vi "PZT Set Position-精调-信号灯.vi"(8 "Set Position （°/mm）":dbl, 9 "Origin":dbl=123.091, 10 "Range":dbl=335.57, 11 "Instrument":T1={"325 Resource "="GPIB0::13::INSTR", "Input (0:A) 325"=0, "Heater Output (1:1) 325"=1, "340 Resource"="GPIB0::14::INSTR", "Input (0:A) 340"=0, "Loop (0: 1)"=0, "Input (0:B) 340"=1, "Loop (1: 1)"=0, "340 Status"=refnum, "Instrument Type"=enum."PPMS-Rotate", "quantum design"=refnum, "semaphore 325"=refnum, "TCP master instance"=refnum, "M24C Resource"="GPIB0::24::INSTR", "4G supply"="GPIB0::24::INSTR", "Temp Status 24C"=refnum, "Temp"=refnum, "9T信号"=refnum, "limit"={"Field limit"=0.0, "Field rate limit"=0.0, "Temp limit"=0.0, "Temp low limit"=0.0, "Temp rate limit "=0.0}, "4g supply status"=refnum, "vi路径"="", "in-plane"="", "out-plane"="", "in-plane signal"=FALSE, "out-plane signal"=FALSE, "in plane 信号"=refnum, "pzt volt"=refnum, "Aborting"=refnum, "数据文件"=refnum, "warning"=refnum, "750 visa"="", "750 rotate"="", "335 Status 2"=refnum, "335 Resource "="GPIB0::24::INSTR", "Input (0:A) 335"=0, "Input (0:B) 335"=1, "Heater Output (1:1) 335"=1, "semaphore 340"=refnum, "semaphore 335"=refnum, "325 Status"=refnum, "semaphore 750"=refnum, "750 field status"=refnum, "camg 振荡状态"=refnum, "列表框"=refnum, "编辑列表框？"=refnum, "camg Rate"=refnum, "行数"=refnum, "TM620"="TCPIP0::192.168.1.5::4266::SOCKET"} {"Loop (1: 1)" items=["1"=1, "2"=2]; "Loop (0: 1)" items=["1"=1, "2"=2]; "Input (0:B) 340" items=["A", "B", "C", "D"]; "Heater Output (1:1) 335" items=["1"=1, "2"=2]; "Input (0:B) 335" items=["A", "B"]; "Input (0:A) 335" items=["A", "B"]; "Heater Output (1:1) 325" items=["1"=1, "2"=2]; "Input (0:A) 325" items=["A", "B"]; "Input (0:A) 340" items=["1"=1, "2"=2]}) -> (1 "Set Position-Real （°/mm）":dbl, 2 "Current Position （mm  /  °）":dbl)   [LabVIEW 2019, in "User lib.lvlib"]
uses:
  User lib.lvlib
  ctl/Instrument.ctl
  <vilib>/NI/Modbus Library/API/Master/Modbus Master.lvclass
  ctl/335 state.ctl
  ctl/Instrument Type.ctl
  C:/Users/fuyang/Desktop/postdoctor/labview/labview-measure/lib/QDInstrument.dll
  lib/QDInstrument.dll
  ctl/limit.ctl
  ctl/9T mag field stauts.ctl
  ctl/warning.ctl
panel:
  out "初始运动方向":bool
  out "x > 0?":bool
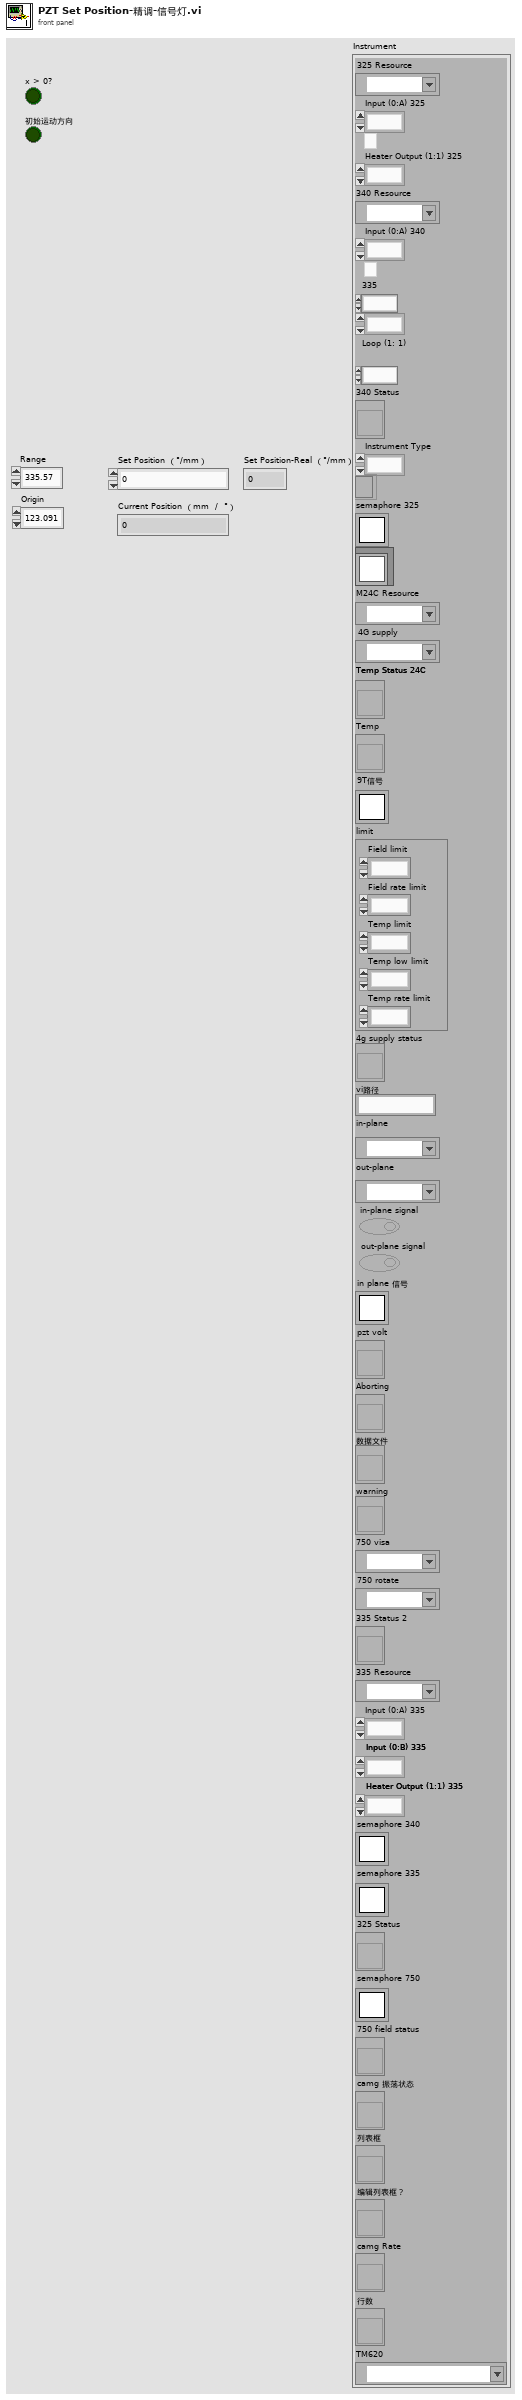
[diagram p1: front panel]
types:
  T1 = typedef "Instrument.ctl" = cluster{"325 Resource ":refnum<visa-resource-name>, "Input (0:A) 325":u16, "Heater Output (1:1) 325":u16, "340 Resource":refnum<visa-resource-name>, "Input (0:A) 340":u16, "Loop (0: 1)":u16, "Input (0:B) 340":u16, "Loop (1: 1)":u16, "340 Status":refnum<vi>, "Instrument Type":T2, "quantum design":refnum<k24>, "semaphore 325":T3, "TCP master instance":refnum<class "Modbus Master.lvclass">, "M24C Resource":refnum<visa-resource-name>, "4G supply":refnum<visa-resource-name>, "Temp Status 24C":refnum<vi>, "Temp":refnum<vi>, "9T信号":T3, "limit":T4, "4g supply status":refnum<vi>, "vi路径":string, "in-plane":refnum<visa-resource-name>, "out-plane":refnum<visa-resource-name>, "in-plane signal":bool, "out-plane signal":bool, "in plane 信号":T3, "pzt volt":refnum<vi>, "Aborting":refnum<vi>, "数据文件":refnum<vi>, "warning":refnum<vi>, "750 visa":refnum<visa-resource-name>, "750 rotate":refnum<visa-resource-name>, "335 Status 2":refnum<vi>, "335 Resource ":refnum<visa-resource-name>, "Input (0:A) 335":u16, "Input (0:B) 335":u16, "Heater Output (1:1) 335":u16, "semaphore 340":T3, "semaphore 335":T3, "325 Status":refnum<vi>, "semaphore 750":T3, "750 field status":refnum<vi>, "camg 振荡状态":refnum<vi>, "列表框":refnum<vi>, "编辑列表框？":refnum<vi>, "camg Rate":refnum<vi>, "行数":refnum<vi>, "TM620":refnum<visa-resource-name>}
  T2 = typedef "Instrument Type.ctl" = enum16{"PPMS", "VersaLab", "DynaCool", "SVSM", "PPMS-Rotate", "Lakeshore335", "lengtou2", "9T mag old", "9T cmag", "9T cmag DAC", "9T cmag rotate", "test"}
  T3 = typedef "Semaphore RefNum" = refnum<k1>
  T4 = typedef "limit.ctl" = cluster{"Field limit":dbl, "Field rate limit":dbl, "Temp limit":dbl, "Temp low limit":dbl, "Temp rate limit ":dbl}
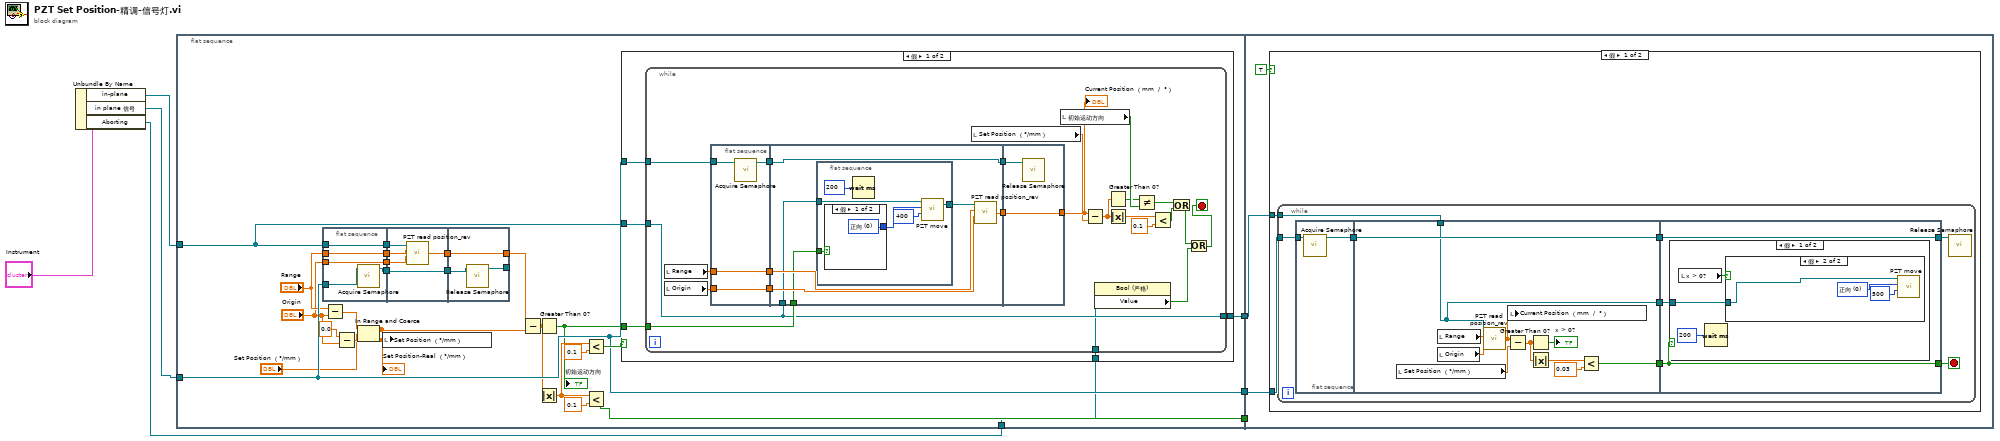
[diagram p0: block diagram]
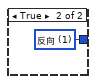
[diagram p2: hidden frame]
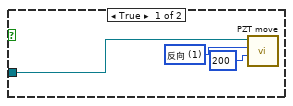
[diagram p4: hidden frame]
diagram:
  n1 = Unbundle By Name("Instrument") -> ("in-plane"=w4:refnum<visa-resource-name>, "in plane 信号"=w2:T3, "Aborting"=w1:refnum<vi>)
  n2 = flat-sequence {
    tunnel: [w31] -> w7
    tunnel: [w30] -> w6
    tunnel: w2 -> [w31]
    tunnel: w4 -> [w10]
    tunnel: [w9] -> w3
    tunnel: w1 -> [w8]
    tunnel: w7 -> [w98]
    tunnel: w6 -> [_]
    tunnel: w3 -> [w96]
    frame #0 {
      n3 = flat-sequence {
        tunnel: "Origin" -> [w35]
        tunnel: "Range" -> [w36]
        tunnel: w10 -> [w37]
        tunnel: [w37] -> w29
        tunnel: [w36] -> w28
        tunnel: [w35] -> w27
        tunnel: w31 -> [w34]
        tunnel: [w33] -> w26
        tunnel: w29 -> [w42]
        tunnel: w28 -> [w40]
        tunnel: w27 -> [w39]
        tunnel: [w41] -> w25
        tunnel: [w38] -> w24
        tunnel: w26 -> [w38]
        tunnel: [w45] -> w23
        tunnel: w25 -> [w45]
        tunnel: w24 -> [w44]
        tunnel: [w43] -> _
        frame #0 {
          n4 = call <vilib>:"Acquire Semaphore.vi"("semaphore"=w34) -> ("semaphore out"=w33:T3)  [unwired: 4 in, 2 out]
        }
        frame #1 {
          n5 = call "PZT read position_rev.vi"("Origin"=w39, "Range"=w40, "VISA resource name"=w42) -> ("Current Position （mm  /  °）"=w41:dbl)  [unwired: 1 in, 2 out]
        }
        frame #2 {
          n6 = call <vilib>:"Release Semaphore.vi"("semaphore"=w44) -> ("semaphore out"=w43:T3)  [unwired: 5 in, 1 out]
        }
      }
      n7 = Subtract(x="Range", y="Origin") -> (x-y=w19:dbl)
      n8 = Subtract(x=0.0, y="Origin") -> (x-y=w18:dbl)
      n9 = In Range and Coerce(upper limit=w19, x="Set Position （°/mm）", lower limit=w18) -> (coerced(x)=w16:dbl)  [unwired: 1 out]
      "Set Position-Real （°/mm）" <- w16
      n10 = local write "Set Position （°/mm）"(w16) -> ()
      n11 = Subtract(x=w23, y=w16) -> (x-y=w21:dbl)
      n12 = Greater Than 0?(x=w21) -> (x > 0?=w11:bool)
      "初始运动方向" <- w11
      n13 = Absolute Value(x=w21) -> (abs(x)=w13:dbl)
      n14 = Less?(x=w13, y=0.1) -> (x < y?=w32:bool)
      n15 = Less?(x=w13, y=0.1) -> (x < y?=w30:bool)
      n16 = case shown="假" w32 {
        tunnel: w31 -> [w50 _]
        tunnel: w11 -> [w49 _]
        tunnel: w10 -> [w48 w95]
        tunnel: [w47 w95] -> w9
        tunnel: w8 -> [w46 _]
        frame False {
          n17 = while {
            tunnel: w50 -> [w57]
            tunnel: w49 -> [w56]
            tunnel: w48 -> [w55]
            tunnel: [w55] -> w47
            tunnel: w46 -> [w54]
            stop <- w51 stop-if-true
            n18 = local read "Range"() -> (w73:dbl)
            n19 = local read "Origin"() -> (w72:dbl)
            n20 = flat-sequence {
              tunnel: w72 -> [w76]
              tunnel: w73 -> [w77]
              tunnel: [w77] -> w61
              tunnel: [w76] -> w60
              tunnel: [w75] -> w58
              tunnel: w57 -> [w74]
              tunnel: [w82] -> w62
              tunnel: w61 -> [w84]
              tunnel: w60 -> [w83]
              tunnel: [w81] -> w59
              tunnel: w58 -> [w81]
              tunnel: w55 -> [w80]
              tunnel: w56 -> [w79]
              tunnel: [w94] -> w71
              tunnel: w62 -> [w94]
              tunnel: w59 -> [w93]
              frame #0 {
                n21 = call <vilib>:"Acquire Semaphore.vi"("semaphore"=w74) -> ("semaphore out"=w75:T3)  [unwired: 4 in, 2 out]
              }
              frame #1 {
                n22 = flat-sequence {
                  tunnel: w80 -> [w90]
                  tunnel: [w88] -> w78
                  tunnel: w79 -> [w87]
                  frame #0 {
                    n23 = case shown="假" w87 {
                      tunnel: [w91 w92] -> w86
                      frame False {
                        w91 = u16 0 items=["正向", "反向"] ("移动方向")
                      }
                      frame True {
                        w92 = u16 1 items=["正向", "反向"] ("移动方向")
                      }
                    }
                    n24 = Wait (ms)(milliseconds to wait=u32 200 ("等待时间（毫秒）")) -> ()  [unwired: 1 out]
                    n25 = call "PZT move.vi"("移动步数"=400, "移动方向"=w86, "VISA resource name"=w90) -> ("VISA资源名称输出"=w88:refnum<visa-resource-name>)  [unwired: 1 in, 1 out]
                  }
                }
                n26 = call "PZT read position_rev.vi"("Origin"=w83, "Range"=w84, "VISA resource name"=w78) -> ("Current Position （mm  /  °）"=w82:dbl)  [unwired: 1 in, 2 out]
              }
              frame #2 {
                n27 = call <vilib>:"Release Semaphore.vi"("semaphore"=w93) -> ()  [unwired: 5 in, 2 out]
              }
            }
            n28 = local read "Set Position （°/mm）"() -> (w70:dbl)
            n29 = local read "初始运动方向"() -> (w66:bool)
            n30 = Subtract(x=w71, y=w70) -> (x-y=w67:dbl)
            n31 = property class="Bool (严格)"(reference=w54) -> ("Value"=w52:bool)  [unwired: 1 in, 2 out]
            n32 = Greater Than 0?(x=w67) -> (x > 0?=w65:bool)
            n33 = Absolute Value(x=w67) -> (abs(x)=w69:dbl)
            n34 = Not Equal?(x=w65, y=w66) -> (x != y?=w64:bool)
            n35 = Less?(x=w69, y=0.1) -> (x < y?=w63:bool)
            n36 = Or(x=w64, y=w63) -> (x .or. y?=w53:bool)
            n37 = Or(x=w53, y=w52) -> (x .or. y?=w51:bool)
            "Current Position （mm  /  °）" <- w71
          }
        }
        frame True {
        }
      }
    }
    frame #1 {
      n38 = case shown="假" TRUE {
        tunnel: w98 -> [w100 _]
        tunnel: w96 -> [w99 _]
        frame False {
          n39 = while {
            tunnel: w100 -> [w107]
            tunnel: w99 -> [w102]
            stop <- w108 stop-if-true
            n40 = flat-sequence {
              tunnel: [w110] -> w106
              tunnel: w107 -> [w109]
              tunnel: [w115] -> w105
              tunnel: w106 -> [w112]
              tunnel: [w112] -> w104
              tunnel: w102 -> [w111]
              tunnel: [w111] -> w101
              tunnel: [w123] -> w108
              tunnel: [w124] -> w103
              tunnel: w104 -> [w124]
              tunnel: w105 -> [w123]
              tunnel: w101 -> [w122]
              frame #0 {
                n41 = call <vilib>:"Acquire Semaphore.vi"("semaphore"=w109) -> ("semaphore out"=w110:T3)  [unwired: 4 in, 2 out]
              }
              frame #1 {
                n42 = local read "Set Position （°/mm）"() -> (w119:dbl)
                n43 = local read "Range"() -> (w121:dbl)
                n44 = local read "Origin"() -> (w120:dbl)
                n45 = call "PZT read position_rev.vi"("Origin"=w120, "Range"=w121, "VISA resource name"=w111) -> ("Current Position （mm  /  °）"=w113:dbl)  [unwired: 1 in, 2 out]
                n46 = Subtract(x=w113, y=w119) -> (x-y=w118:dbl)
                n47 = local write "Current Position （mm  /  °）"(w113) -> ()
                n48 = Greater Than 0?(x=w118) -> (x > 0?=→"x > 0?":bool)
                n49 = Absolute Value(x=w118) -> (abs(x)=w117:dbl)
                n50 = Less?(x=w117, y=0.03) -> (x < y?=w115:bool)
              }
              frame #2 {
                n51 = case shown="假" w123 {
                  tunnel: w122 -> [w125 _]
                  frame False {
                    n52 = local read "x > 0?"() -> (w127:bool)
                    n53 = Wait (ms)(milliseconds to wait=u32 200) -> ()  [unwired: 1 out]
                    n54 = case shown="假" w127 {
                      tunnel: w125 -> [w128 w131]
                      frame True {
                        w130 = u16 1 items=["正向", "反向"] ("移动方向")
                        n55 = call "PZT move.vi"("移动步数"=200, "移动方向"=w130, "VISA resource name"=w128) -> ()  [unwired: 1 in, 2 out]
                      }
                      frame False {
                        w133 = u16 0 items=["正向", "反向"] ("移动方向")
                        n56 = call "PZT move.vi"("移动步数"=500, "移动方向"=w133, "VISA resource name"=w131) -> ()  [unwired: 1 in, 2 out]
                      }
                    }
                  }
                  frame True {
                  }
                }
              }
            }
            n57 = call <vilib>:"Release Semaphore.vi"("semaphore"=w103) -> ()  [unwired: 5 in, 2 out]
          }
        }
        frame True {
        }
      }
    }
  }
